vi "Abort.vi"(4 "Function":enum16{"Read", "Write"}(ring), 6 "Abort":bool, 7 "Error In":errorcluster) -> (1 "Abort out":bool, 2 "Error Out":errorcluster)   [LabVIEW 2014]
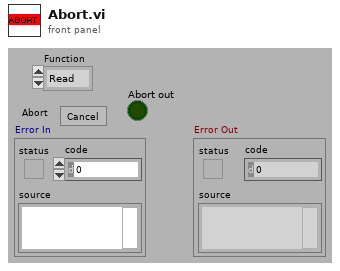
[diagram p1: front panel]
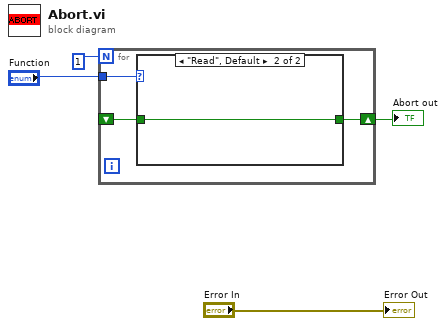
[diagram p0: block diagram]
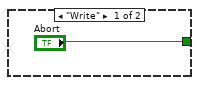
[diagram p2: hidden frame]
diagram:
  n1 = for {
    N: 1 -> [_]
    shift-right: [w6] -> w3
    shift-left: _ -> [w7]
    tunnel: "Function" -> [w5]
    n2 = case shown="\"Read\", Default" w5 {
      tunnel: w7 -> [_ w9]
      tunnel: ["Abort" w9] -> w6
      frame "Write" {
      }
      frame "Read", Default {
      }
    }
  }
  "Abort out" <- w3
  "Error Out" <- "Error In"
